vi "Fgen Arb Tester (SS-OCT)_Ascan.vi"() -> ()   [LabVIEW 2012]
doc: "This example shows how to use the Arbitrary Waveform mode to generate on two channels."
uses:
  <instrlib>/niFgen/niFgen.llb/niFgen Output Mode.ctl
  <instrlib>/niFgen/niFgen.llb/niFgen Write Waveform.vi
panel:
  in  "OCT Signal":path=path "C:/Users/kvemishe/Documents/K-Trigger Data/Jesung Data/A&M_OCTdata_12292011/finger_bscan_2_OCT1.bin"
  in  "Reference Signal":path=path "C:/Users/kvemishe/Documents/K-Trigger Data/Jesung Data/A&M_OCTdata_12292011/finger_bscan_2_OCT2.bin"
  in  "CH1 Gain":dbl(knob)=1.0 caption="CH 1 Gain" step=0.0001 scale=0.0..2.5 scale format="%#.7f"
  out "Graph":dbl[][](graph)
  in  "CH0 Gain":dbl(knob)=1.0 caption="CH 0 Gain" step=0.0001 scale=0.0..2.5 scale format="%#.7f"
  in  "Sample Rate":dbl=250000000.0 format="%.2p"
  in  "stop":bool
  in  "Update":bool
  in  "Sample Clock Source":string(combo)="OnboardClock"
  in  "Resource Name":refnum<k15>="5451"
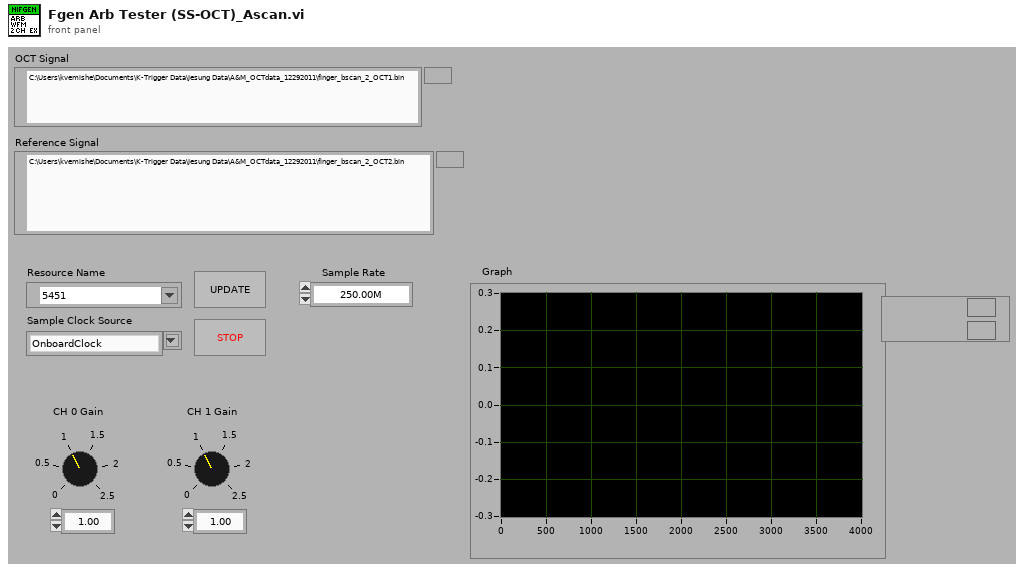
[diagram p1: front panel]
types:
  T1 = typedef "niFgen Output Mode.ctl" = u32
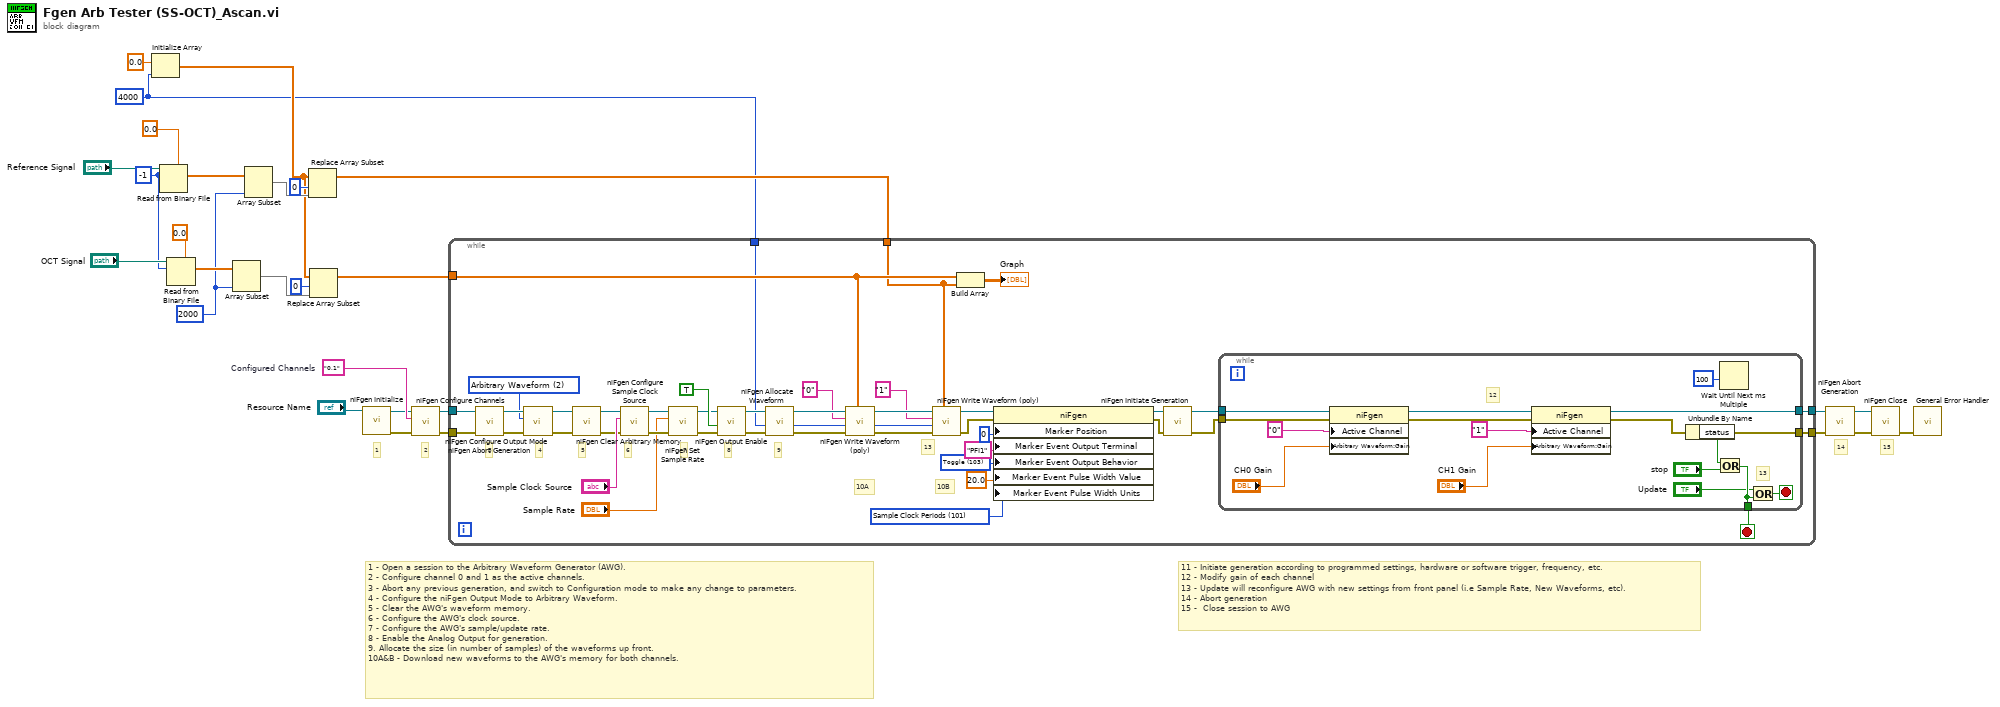
[diagram p0: block diagram]
diagram:
  w1 = 4000 ("dimension size")
  w4 = 2000 ("length")
  w13 = -1 ("count (1)")
  w22 = "0,1"  # Configured Channels
  # "15"
  # "11 - Initiate generation according to programmed settings, hardware or software trigger, frequency, etc.\n12 - Modify gain of each channel \n13 - Update will reconfigure AWG with new settings from front panel (i.e Sample Rate, New Waveforms, etc).\n14 - Abort generation\n15 -  Close session to AWG"
  # "2"
  # "14"
  # "1"
  # "1 - Open a session to the Arbitrary Waveform Generator (AWG).\n2 - Configure channel 0 and 1 as the active channels.\n3 - Abort any previous generation, and switch to Configuration mode to make any change to parameters.\n4 - Configure the niFgen Output Mode to Arbitrary Waveform.\n5 - Clear the AWG's waveform memory.\n6 - Configure the AWG's clock source.\n7 - Configure the AWG's sample/update rate.\n8 - Enable the Analog Output for generation.\n9. Allocate the size (in number of samples) of the waveforms up front.\n10A&B - Download new waveforms to the AWG's memory for both channels."
  n1 = Initialize Array(0.0 ("element"), w1) -> (w5:dbl[])
  n2 = Read from Binary File(5:0.0, 10:w13, 11:"Reference Signal") -> (2:w12:dbl[])  [unwired: 3 in, 3 out]
  n3 = Read from Binary File(5:0.0, 10:w13, 11:"OCT Signal") -> (2:w11:dbl[])  [unwired: 3 in, 3 out]
  n4 = Array Subset(array=w11, length=w4) -> (w8:dbl[])  [unwired: 1 in]
  n5 = Array Subset(array=w12, length=w4) -> (w9:dbl[])  [unwired: 1 in]
  n6 = Replace Array Subset(array=w5, new element=w9, index=0) -> (w2:dbl[])
  n7 = Replace Array Subset(array=w5, new element=w8, index=0) -> (w3:dbl[])
  n8 = call <instrlib>:"niFgen Initialize.vi"("Resource Name"="Resource Name") -> ("error out"=w21:errorcluster, "Instrument Handle Out"=w18:refnum<k15>)  [unwired: 3 in, 6 out]
  n9 = call <instrlib>:"niFgen Configure Channels.vi"("error in (no error)"=w21, "Channels"=w22, "Instrument Handle"=w18) -> ("error out"=w20:errorcluster, "Instrument Handle Out"=w19:refnum<k15>)  [unwired: 7 out]
  n10 = while {
    tunnel: [w59] -> w27
    tunnel: [w71] -> w28
    tunnel: w20 -> [w61]
    tunnel: w19 -> [w70]
    tunnel: w3 -> [w40]
    tunnel: w2 -> [w39]
    tunnel: w1 -> [w38]
    stop <- w72 stop-if-true
    w30 = 101 items=["Sample Clock Periods"=101, "Seconds"=102] ("Events:Marker:Pulse:Width Units")
    w31 = 103 items=["Pulse"=101, "Toggle"=103] ("Events:Marker:Output Behavior")
    w67 = T1 2 items=["Standard Function", "Frequency List", "Arbitrary Waveform", "Arbitrary Sequence", "Script"] ("Output Mode")
    # "11"
    # "10B"
    # "13"
    # "8"
    # "7"
    # "6"
    # "10A"
    # "9"
    # "5"
    # "4"
    # "3"
    n11 = call <instrlib>:"niFgen Abort Generation.vi"("error in (no error)"=w61, "Instrument Handle"=w70) -> ("error out"=w69:errorcluster, "Instrument Handle Out"=w68:refnum<k15>)  [unwired: 8 out]
    n12 = call <instrlib>:"niFgen Configure Output Mode.vi"("error in (no error)"=w69, "Output Mode (default: 0=Standard Function)"=w67, "Instrument Handle"=w68) -> ("error out"=w65:errorcluster, "Instrument Handle Out"=w66:refnum<k15>)  [unwired: 6 out]
    n13 = call <instrlib>:"niFgen Clear Arbitrary Memory.vi"("error in (no error)"=w65, "Instrument Handle"=w66) -> ("error out"=w45:errorcluster, "Instrument Handle Out"=w46:refnum<k15>)  [unwired: 8 out]
    n14 = call <instrlib>:"niFgen Configure Sample Clock Source.vi"("error in (no error)"=w45, "Source (Onboard Clock)"="Sample Clock Source", "Instrument Handle"=w46) -> ("error out"=w63:errorcluster, "Instrument Handle Out"=w64:refnum<k15>)  [unwired: 7 out]
    n15 = call <instrlib>:"niFgen Set Sample Rate.vi"("error in (no error)"=w63, "Sample Rate (Samp/s)"="Sample Rate", "Instrument Handle"=w64) -> ("error out"=w43:errorcluster, "Instrument Handle Out"=w44:refnum<k15>)  [unwired: 7 out]
    n16 = call <instrlib>:"niFgen Output Enable.vi"("error in (no error)"=w43, "Output Enable (default: True)"=TRUE ("output enable"), "Instrument Handle"=w44) -> ("error out"=w52:errorcluster, "Instrument Handle Out"=w51:refnum<k15>)  [unwired: 1 in, 6 out]
    n17 = call <instrlib>:"niFgen Allocate Waveform.vi"("error in (no error)"=w52, "Waveform Size"=w38, "Instrument Handle"=w51) -> ("error out"=w50:errorcluster, "Waveform Handle Out"=w53:i32, "Instrument Handle Out"=w49:refnum<k15>)  [unwired: 1 in, 5 out]
    n18 = call-poly <instrlib>:"niFgen Write Waveform (poly).vi"("Waveform Data"=w40, "error in (no error)"=w50, "Waveform Handle"=w53, "Channel Name"="0", "Instrument Handle"=w49) -> ("error out"=w56:errorcluster, "Waveform Handle Out"=w54:i32, "Instrument Handle Out"=w55:refnum<k15>)  [unwired: 4 out]
    n19 = call-poly <instrlib>:"niFgen Write Waveform (poly).vi"("Waveform Data"=w39, "error in (no error)"=w56, "Waveform Handle"=w54, "Channel Name"="1", "Instrument Handle"=w55) -> ("error out"=w36:errorcluster, "Instrument Handle Out"=w37:refnum<k15>)  [unwired: 5 out]
    n20 = Build Array(w40, w39) -> (→"Graph":dbl[][])
    n21 = property class="niFgen"(reference=w37, error in=w36, "Marker Position"=0 ("Arbitrary Waveform:Arbitrary Waveform Mode:Marker Position"), "Marker Event Output Terminal"="PFI1" ("Events:Marker:Output Terminal"), "Marker Event Output Behavior"=w31, "Marker Event Pulse Width Value"=20.0 ("Events:Marker:Pulse:Width Value"), "Marker Event Pulse Width Units"=w30) -> (reference out=w35:refnum<k15>, error out=w34:errorcluster)
    n22 = call <instrlib>:"niFgen Initiate Generation.vi"("error in (no error)"=w34, "Instrument Handle"=w35) -> ("error out"=w41:errorcluster, "Instrument Handle Out"=w42:refnum<k15>)  [unwired: 8 out]
    n23 = while {
      tunnel: [w73] -> w71
      tunnel: w42 -> [w82]
      tunnel: [w84] -> w72
      tunnel: w41 -> [w81]
      tunnel: [w74] -> w59
      stop <- w87 stop-if-true
      # "12"
      # "13"
      n24 = property class="niFgen"(reference=w82, error in=w81, "Active Channel"="0", "Arbitrary Waveform:Gain"="CH0 Gain") -> (reference out=w78:refnum<k15>, error out=w77:errorcluster)
      n25 = property class="niFgen"(reference=w78, error in=w77, "Active Channel"="1", "Arbitrary Waveform:Gain"="CH1 Gain") -> (reference out=w73:refnum<k15>, error out=w74:errorcluster)
      n26 = Unbundle By Name(w74) -> ("status"=w85:bool)
      n27 = Or(x=w85, y="stop") -> (x .or. y?=w84:bool)
      n28 = Wait Until Next ms Multiple(millisecond multiple=u32 100) -> ()  [unwired: 1 out]
      n29 = Or(x="Update", y=w84) -> (x .or. y?=w87:bool)
    }
  }
  n30 = call <instrlib>:"niFgen Abort Generation.vi"("error in (no error)"=w27, "Instrument Handle"=w28) -> ("error out"=w26:errorcluster, "Instrument Handle Out"=w25:refnum<k15>)  [unwired: 8 out]
  n31 = call <instrlib>:"niFgen Close.vi"("error in (no error)"=w26, "Instrument Handle"=w25) -> ("error out"=w23:errorcluster)  [unwired: 9 out]
  n32 = call <vilib>:"General Error Handler.vi"("error in (no error)"=w23) -> ()  [unwired: 1 in, 14 out]
